vi "Run Config Data Encoder.vi"(10 "uS array":string[](array[string]), 11 "Run Config Name":string) -> (3 "Run config data array":string[](array[string]))   [LabVIEW 2026, in "TALOS.lvlib" / "Guardian.lvlib" / "Guardian.lvclass"]
uses:
  Guardian.lvclass
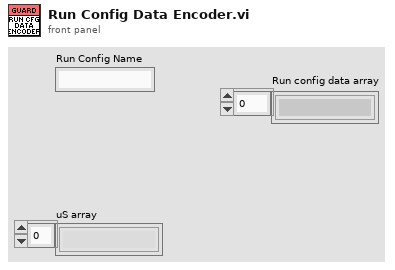
[diagram p1: front panel]
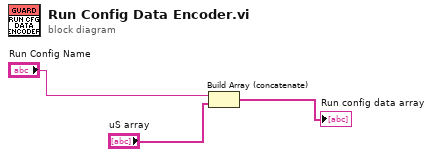
[diagram p0: block diagram]
diagram:
  n1 = Build Array (concatenate)("Run Config Name", "uS array") -> (→"Run config data array":string[])
